vi "CloseFile.vi"(8 "error in (no error)":errorcluster, 11 "TrigBoxINIFileClass in":refnum<class "TrigBoxINIFileClass.lvclass">) -> (0 "error out":errorcluster, 3 "TrigBoxINIFileClass out":refnum<class "TrigBoxINIFileClass.lvclass">)   [LabVIEW 2013, in "TrigBoxINIFileClass.lvclass"]
uses:
  TrigBoxINIFileClass.lvclass
  INIFileClass/INIFileClass.lvclass
panel:
  out "AllKeysFound?":bool
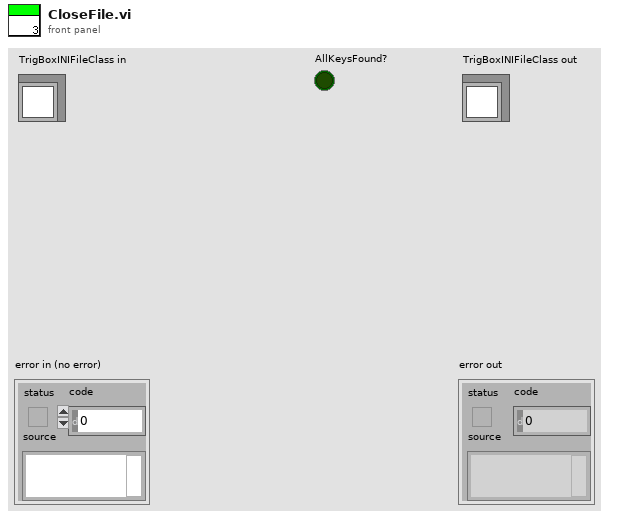
[diagram p1: front panel]
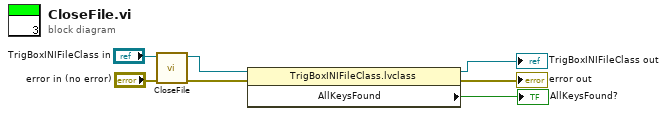
[diagram p0: block diagram]
diagram:
  n1 = call-parent "CloseFile.vi"("error in (no error)"="error in (no error)", "INIFileClass in"="TrigBoxINIFileClass in") -> ("error out"=w4:errorcluster, "INIFileClass out"=w5:refnum<class "TrigBoxINIFileClass.lvclass">)  [unwired: 8 in]
  n2 = property class="TrigBoxINIFileClass.lvclass"(reference=w5, error in=w4) -> (reference out=→"TrigBoxINIFileClass out":refnum<class "TrigBoxINIFileClass.lvclass">, error out=→"error out":errorcluster, "AllKeysFound"=→"AllKeysFound?":bool)
